vi "Polling Core.vi"(8 "Error In":errorcluster, 11 "KIT-QVA in":refnum<class "KIT-QVA.lvclass">) -> (0 "Error Out":errorcluster, 3 "KIT-QVA out":refnum<class "KIT-QVA.lvclass">)   [LabVIEW 2016, in "KIT-QVA.lvlib" / "KIT-QVA.lvclass"]
doc: "Implement the pseudo-periodic action in your override.vi."
uses:
  KIT-QVA.lvclass
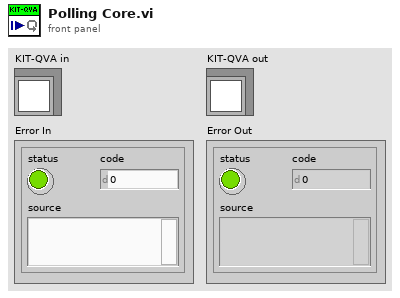
[diagram p1: front panel]
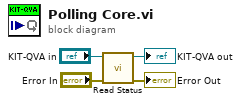
[diagram p0: block diagram]
diagram:
  n1 = call "Read Status.vi"("Error In"="Error In", "KIT-QVA in"="KIT-QVA in") -> ("Error Out"=→"Error Out":errorcluster, "KIT-QVA out"=→"KIT-QVA out":refnum<class "KIT-QVA.lvclass">)  [unwired: 8 in]
